vi "PDHydra Waveform Analysis.vi"(8 "Waveform":waveform(dbl)[](array[waveform])) -> (1 "Frequency":dbl[](array[numeric]), 2 "RMS values":dbl[](array[numeric]) format="%.2p", 3 "DC values":dbl[](array[numeric]) format="%.2p")   [LabVIEW 2022 SP3]
uses:
  <vilib>/measure/madcrms.llb/Basic Averaged DC-RMS for N Chan.vi
  <vilib>/measure/mascope.llb/Pulse Measurements N chan.vi
  <vilib>/measure/NI_MAPro.lvlib
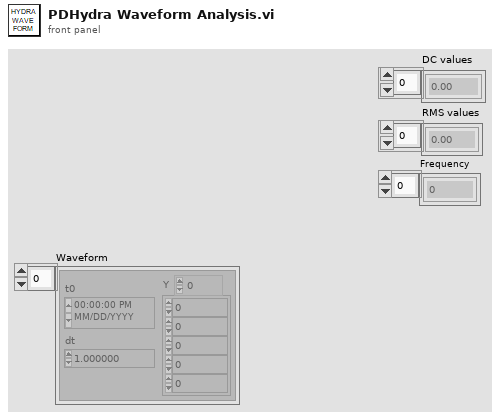
[diagram p1: front panel]
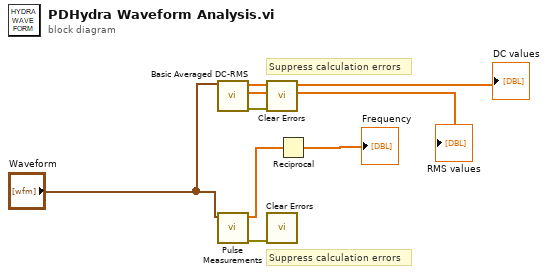
[diagram p0: block diagram]
diagram:
  # "Suppress calculation errors"
  # "Suppress calculation errors"
  n1 = call-poly <vilib>:"Basic Averaged DC-RMS.vi"("signals in"="Waveform") -> ("error out"=w5:errorcluster, "RMS values"=→"RMS values":dbl[], "DC values"=→"DC values":dbl[])  [unwired: 7 in, 1 out]
  n2 = call-poly <vilib>:"Pulse Measurements.vi"("signal(s) in"="Waveform") -> ("error out"=w6:errorcluster, "period"=w7:dbl[])  [unwired: 6 in, 3 out]
  n3 = call <vilib>:"Clear Errors.vi"("error in (no error)"=w5) -> ()  [unwired: 5 in, 2 out]
  n4 = call <vilib>:"Clear Errors.vi"("error in (no error)"=w6) -> ()  [unwired: 5 in, 2 out]
  n5 = Reciprocal(x=w7) -> (1/x=→"Frequency":dbl[])
